vi "Loading Ascan data.vi"(8 "error in (no error)":errorcluster caption="错误输入（无错误）", 11 "名称或相对路径":string) -> (0 "error out":errorcluster caption="错误输出", 3 "first row":dbl[](array[numeric]) caption="第一行")   [LabVIEW 2015, in "Utility VIs.lvlib"]
uses:
  Utility VIs.lvlib
  <vilib>/Utility/file.llb/Read Delimited Spreadsheet (DBL).vi
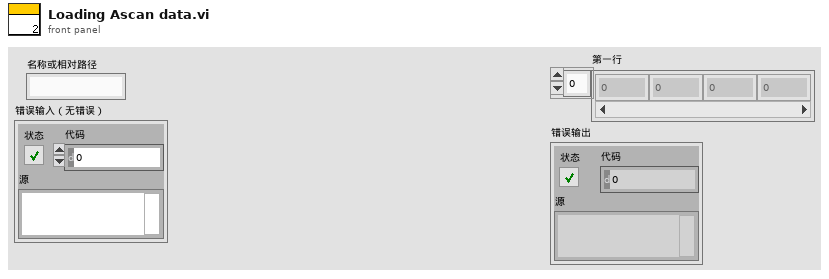
[diagram p1: front panel]
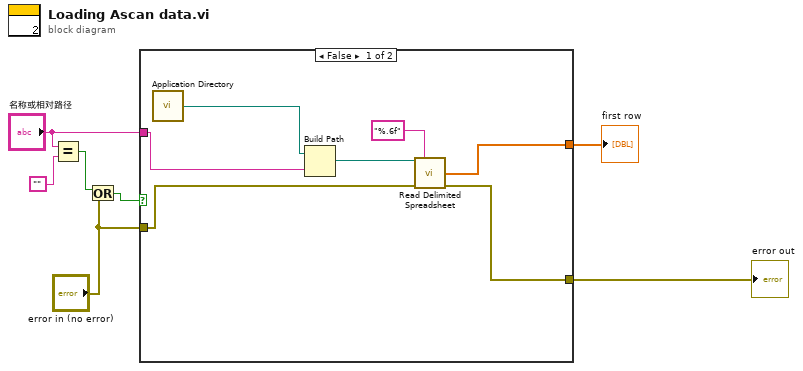
[diagram p0: block diagram]
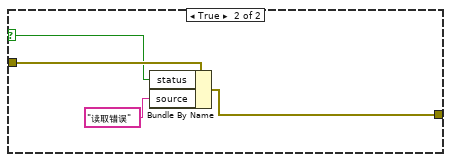
[diagram p2: hidden frame]
diagram:
  n1 = Equal?(x="名称或相对路径", y="") -> (x = y?=w4:bool)
  n2 = Or(x=w4, y="error in (no error)") -> (x .or. y?=w3:bool)
  n3 = case shown="False" w3 {
    selector: w3 -> [_ w17]
    tunnel: [w12 _] -> w7
    tunnel: [w11 w15] -> w6
    tunnel: "名称或相对路径" -> [w10 _]
    tunnel: "error in (no error)" -> [w9 w18]
    frame False {
      n4 = call <vilib>:"Application Directory.vi"() -> ("Application Directory"=w14:path)
      n5 = Build Path(base path=w14, name or relative path=w10) -> (appended path=w13:path)
      n6 = call-poly <vilib>:"Read Delimited Spreadsheet.vi"("file path (dialog if empty)"=w13, "format (%.3f)"="%.6f", "error in (no error)"=w9) -> ("first row"=w12:dbl[], "error out"=w11:errorcluster)  [unwired: 7 in, 4 out]
    }
    frame True {
      n7 = Bundle By Name(cluster=w18, "status"=w17, "source"="读取错误") -> (w15:errorcluster)
    }
  }
  "first row" <- w7
  "error out" <- w6
